vi "Inspection Status_MI.vi"(8 "error in (no error)":errorcluster, 10 "Inspection Status":string(combo), 11 "Machine Interface Actor in":refnum<class "Machine Interface.lvclass">) -> (0 "error out":errorcluster, 3 "Machine Interface Actor out":refnum<class "Machine Interface.lvclass">)   [LabVIEW 2019, in "Machine Interface.lvclass"]
uses:
  Machine Interface.lvclass
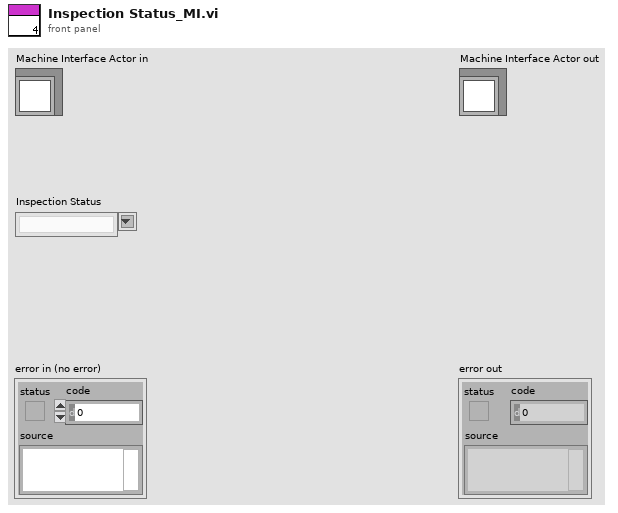
[diagram p1: front panel]
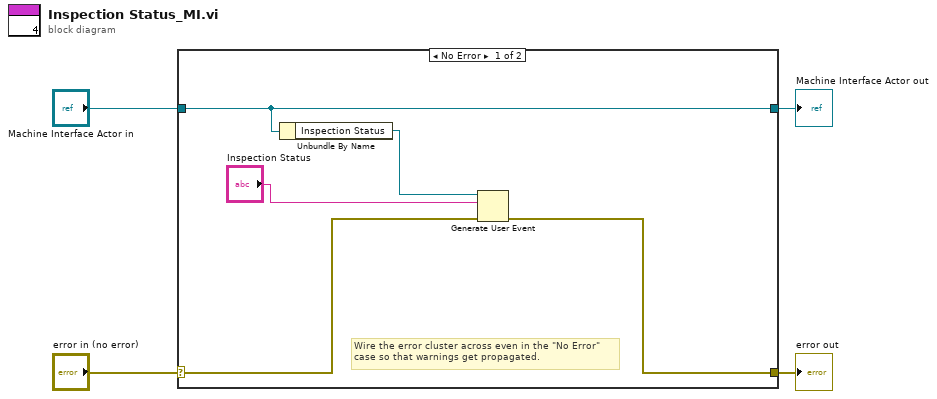
[diagram p0: block diagram]
diagram:
  n1 = case shown="No Error" "error in (no error)" {
    selector: "error in (no error)" -> [w9 w11]
    tunnel: [w8 w11] -> w3
    tunnel: [w6 w10] -> w1
    tunnel: "Machine Interface Actor in" -> [w6 w10]
    frame No Error {
      # "Wire the error cluster across even in the \"No Error\"\ncase so that warnings get propagated."
      n2 = Unbundle By Name(w6) -> ("Inspection Status"=w5:refnum<user-event>)
      n3 = Generate User Event(user event=w5, event data cluster="Inspection Status", error in=w9) -> (error out=w8:errorcluster)  [unwired: 1 in, 1 out]
    }
    frame Error {
    }
  }
  "error out" <- w3
  "Machine Interface Actor out" <- w1
